vi "Get_Response_Type.vi"(8 "error in (no error)":errorcluster, 11 "OneNote in":refnum<class "OneNote.lvclass">) -> (0 "error out":errorcluster, 3 "OneNote out":refnum<class "OneNote.lvclass">)   [LabVIEW 2016, in "OneNote.lvclass"]
uses:
  OneNote.lvclass
  OneNote.lvclass/OneNote.ctl
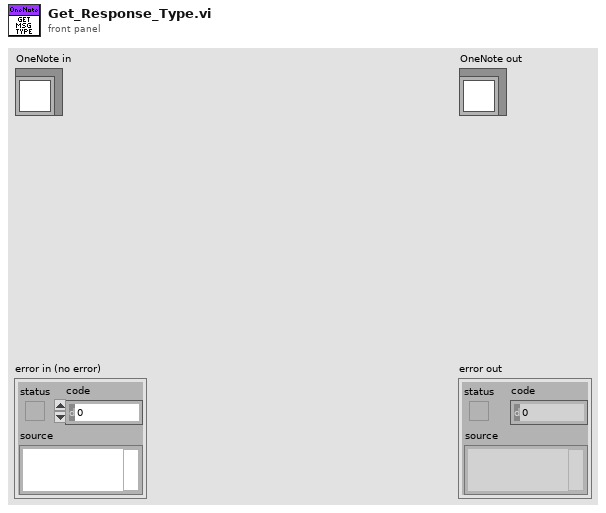
[diagram p1: front panel]
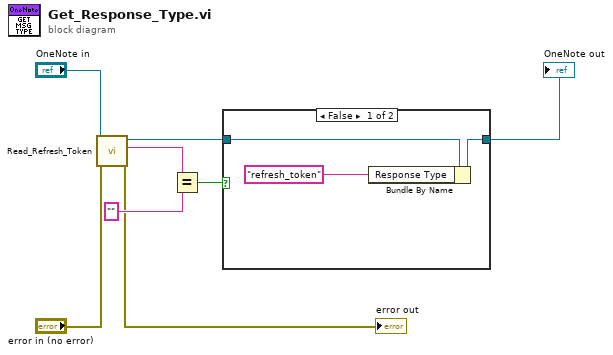
[diagram p0: block diagram]
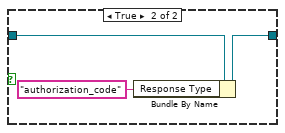
[diagram p2: hidden frame]
diagram:
  n1 = call-dynamic "Read_Refresh_Token.vi"("error in (no error)"="error in (no error)", "OneNote in"="OneNote in") -> ("error out"=→"error out":errorcluster, "String"=w3:string, "OneNote out"=w5:refnum<class "OneNote.lvclass">)  [unwired: 7 in]
  n2 = Equal?(x=w3, y="") -> (x = y?=w8:bool)
  n3 = case shown="False" w8 {
    tunnel: [w11 w14] -> w4
    tunnel: w5 -> [w9 w12]
    frame False {
      n4 = Bundle By Name(cluster=w9, "Response Type"="refresh_token") -> (w11:refnum<class "OneNote.lvclass">)
    }
    frame True {
      n5 = Bundle By Name(cluster=w12, "Response Type"="authorization_code") -> (w14:refnum<class "OneNote.lvclass">)
    }
  }
  "OneNote out" <- w4
